vi "piezoDoubleWriteWriteFuncGen.vi"() -> (0 "success":bool)   [LabVIEW 2017]
doc: "Starts the piezo with a triangle or sine wave in continuous mode."
uses:
  <vilib>/DAQmx/write.llb/DAQmx Write (Analog 2D DBL NChan NSamp).vi
  globalDevices.vi
  globalUtilities.vi
  <vilib>/DAQmx/miscellaneous.llb/DAQmx Fill In Error Info.vi
panel:
  out "offset":dbl
  out "amplitude":dbl
  out "omega":dbl
  out "dt":dbl
  out "nT":i32
  out "Waveform Graph 4":dbl[](graph)
  out "Waveform Graph 3":dbl[](graph)
  out "used dt 2":dbl
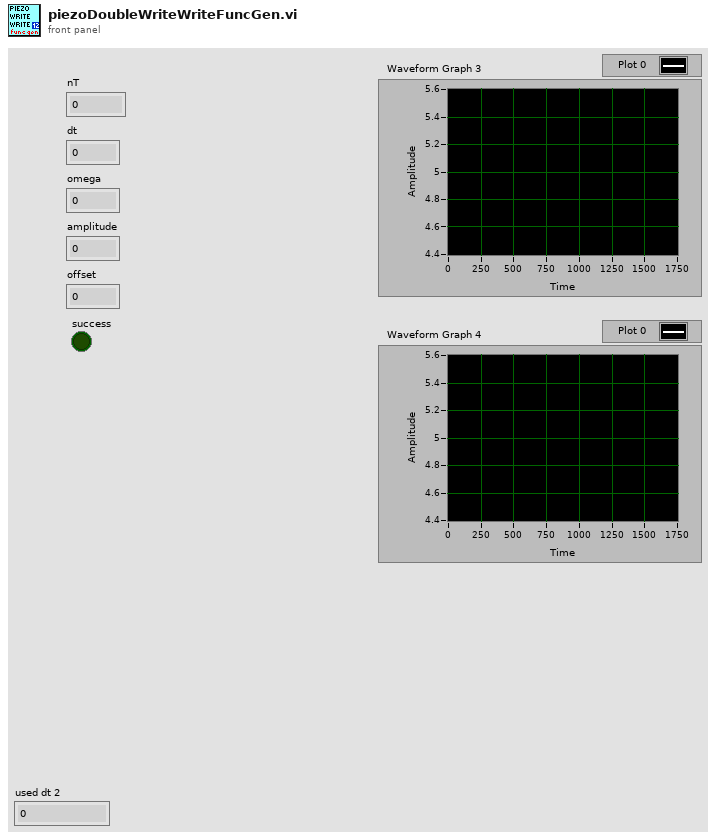
[diagram p1: front panel]
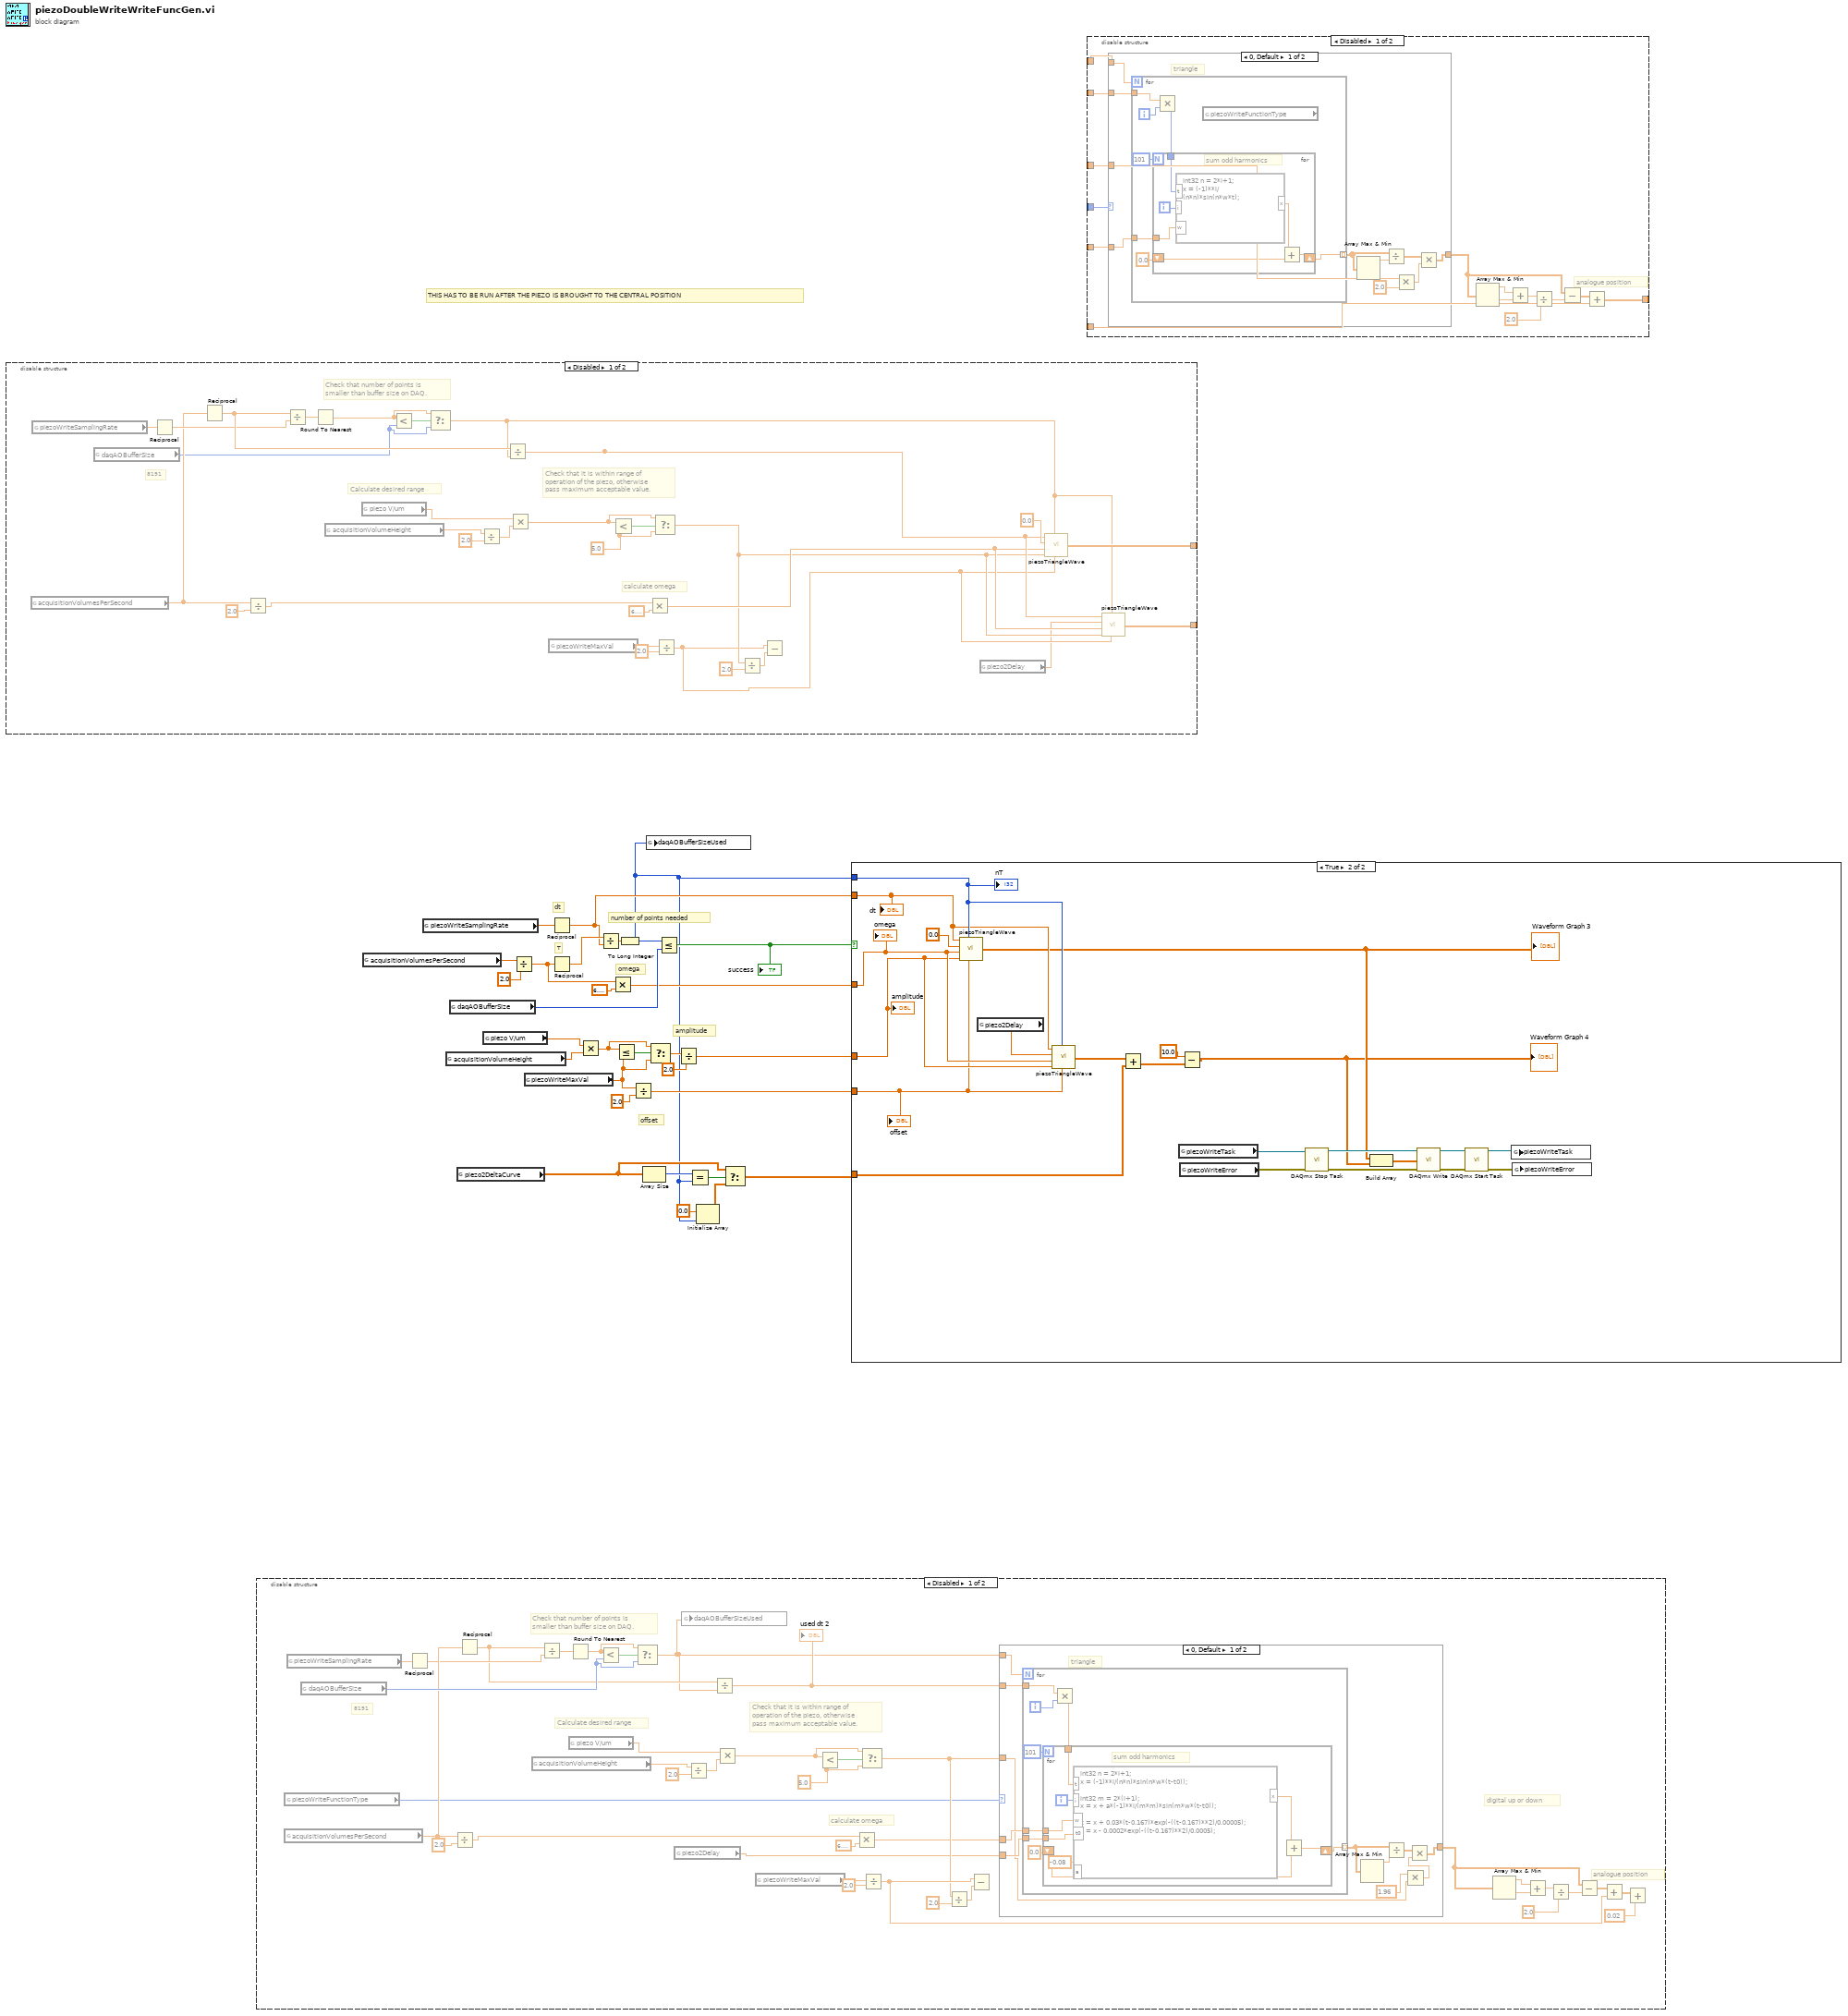
[diagram p0: block diagram]
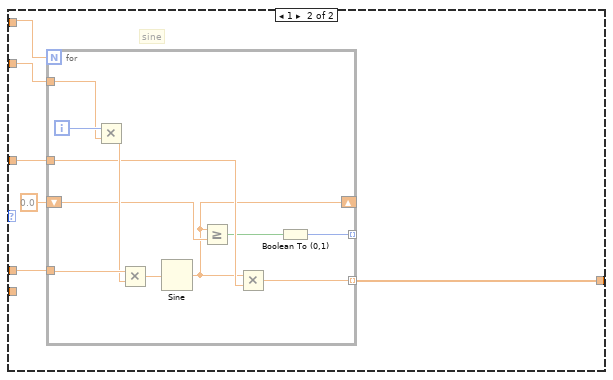
[diagram p4: hidden frame]
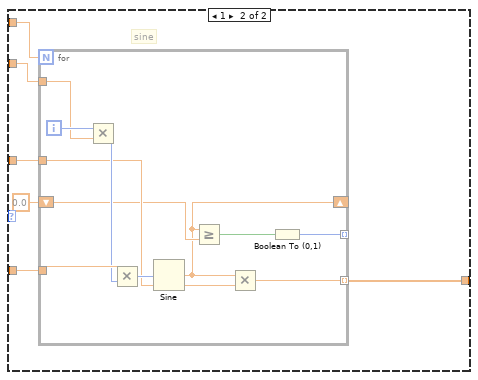
[diagram p6: hidden frame]
diagram:
  # "omega"
  # "amplitude"
  # "offset"
  # "number of points needed"
  # "T"
  # "dt"
  # "THIS HAS TO BE RUN AFTER THE PIEZO IS BROUGHT TO THE CENTRAL POSITION"
  n1 = disable-structure shown="Disabled" {
    disable-tunnel: [w38 _] -> _
    disable-tunnel: [w30 _] -> _
    frame Disabled {
      w53 = 5.0 ("y")
      # "8191"
      # "calculate omega"
      # "Check that number of points is\nsmaller than buffer size on DAQ."
      # "Check that it is within range of\noperation of the piezo, otherwise\npass maximum acceptable value."
      # "Calculate desired range"
      n2 = global read "globalUtilities.vi" "acquisitionVolumesPerSecond"() -> (w44:dbl)
      n3 = global read "globalDevices.vi" "piezoWriteSamplingRate"() -> (w48:dbl)
      n4 = global read "globalDevices.vi" "daqAOBufferSize"() -> (w41:i32)
      n5 = Reciprocal(x=w48) -> (1/x=w47:dbl)
      n6 = Reciprocal(x=w44) -> (1/x=w49:dbl)
      n7 = Divide(x=w44, y=2.0) -> (x/y=w42:dbl)
      n8 = Divide(x=w49, y=w47) -> (x/y=w51:dbl)
      n9 = Round To Nearest(number=w51) -> (nearest integer value=w29:dbl)
      n10 = global read "globalUtilities.vi" "acquisitionVolumeHeight"() -> (w58:dbl)
      n11 = global read "globalDevices.vi" "piezo V/um"() -> (w59:dbl)
      n12 = Less?(x=w29, y=w41) -> (x < y?=w50:bool)
      n13 = Select(t=w29, s=w50, f=w41) -> (s? t:f=w36:dbl)
      n14 = Divide(x=w58, y=2.0) -> (x/y=w56:dbl)
      n15 = Divide(x=w49, y=w36) -> (x/y=w35:dbl)
      n16 = Multiply(x=w59, y=w56) -> (x*y=w54:dbl)
      n17 = global read "globalDevices.vi" "piezoWriteMaxVal"() -> (w46:dbl)
      n18 = Less?(x=w54, y=w53) -> (x < y?=w55:bool)
      n19 = Multiply(x=w42, y=6.283185307179586) -> (x*y=w34:dbl)
      n20 = Select(t=w54, s=w55, f=w53) -> (s? t:f=w33:dbl)
      n21 = Divide(x=w46, y=2.0) -> (x/y=w32:dbl)
      n22 = Divide(x=w33, y=2.0) -> (x/y=w40:dbl)
      n23 = Subtract(x=w32, y=w40) -> ()  [unwired: 1 out]
      n24 = global read "globalDevices.vi" "piezo2Delay"() -> (w31:dbl)
      n25 = call "piezoTriangleWave.vi"("offset"=w32, "nT"=w36, "amplitude"=w33, "omega"=w34, "t0"=0.0, "dt"=w35) -> ("x+y"=w38:dbl[])
      n26 = call "piezoTriangleWave.vi"("offset"=w32, "nT"=w36, "amplitude"=w33, "omega"=w34, "t0"=w31, "dt"=w35) -> ("x+y"=w30:dbl[])
    }
    frame Enabled {
    }
  }
  n27 = disable-structure shown="Disabled" {
    frame Disabled {
      w70 = 5.0 ("y")
      # "8191"
      # "analogue position"
      # "digital up or down"
      # "calculate omega"
      # "Check that number of points is\nsmaller than buffer size on DAQ."
      # "Check that it is within range of\noperation of the piezo, otherwise\npass maximum acceptable value."
      # "Calculate desired range"
      n28 = global read "globalDevices.vi" "piezoWriteFunctionType"() -> (w82:u16)
      n29 = global read "globalUtilities.vi" "acquisitionVolumesPerSecond"() -> (w83:dbl)
      n30 = global read "globalDevices.vi" "piezoWriteSamplingRate"() -> (w78:dbl)
      n31 = global read "globalDevices.vi" "daqAOBufferSize"() -> (w86:i32)
      n32 = Reciprocal(x=w78) -> (1/x=w79:dbl)
      n33 = Divide(x=w83, y=2.0) -> (x/y=w85:dbl)
      n34 = Reciprocal(x=w83) -> (1/x=w76:dbl)
      n35 = global read "globalUtilities.vi" "acquisitionVolumeHeight"() -> (w65:dbl)
      n36 = Divide(x=w76, y=w79) -> (x/y=w73:dbl)
      n37 = Round To Nearest(number=w73) -> (nearest integer value=w75:dbl)
      n38 = global read "globalDevices.vi" "piezo V/um"() -> (w64:dbl)
      n39 = Less?(x=w75, y=w86) -> (x < y?=w74:bool)
      n40 = Select(t=w75, s=w74, f=w86) -> (s? t:f=w60:dbl)
      n41 = global read "globalDevices.vi" "piezo2Delay"() -> (w63:dbl)
      n42 = global write "globalDevices.vi" "daqAOBufferSizeUsed"(w60) -> ()
      n43 = Divide(x=w65, y=2.0) -> (x/y=w67:dbl)
      n44 = Divide(x=w76, y=w60) -> (x/y=w77:dbl)
      "used dt 2" <- w77
      n45 = Multiply(x=w64, y=w67) -> (x*y=w69:dbl)
      n46 = global read "globalDevices.vi" "piezoWriteMaxVal"() -> (w80:dbl)
      n47 = Less?(x=w69, y=w70) -> (x < y?=w68:bool)
      n48 = Multiply(x=w85, y=6.283185307179586) -> (x*y=w72:dbl)
      n49 = Select(t=w69, s=w68, f=w70) -> (s? t:f=w88:dbl)
      n50 = Divide(x=w80, y=2.0) -> (x/y=w97:dbl)
      n51 = Divide(x=w88, y=2.0) -> (x/y=w87:dbl)
      n52 = Subtract(x=w97, y=w87) -> ()  [unwired: 1 out]
      n53 = case shown="0, Default" w82 {
        tunnel: w72 -> [w106 w130]
        tunnel: w60 -> [w108 w129]
        tunnel: w77 -> [w107 w128]
        tunnel: w88 -> [w101 w127]
        tunnel: [w98 w125] -> w95
        tunnel: w63 -> [w105 _]
        frame 0, Default {
          # "triangle"
          n54 = for {
            N: w108 -> [_]
            tunnel: w107 -> [w116]
            tunnel: w106 -> [w113]
            tunnel: [w109] -> w102 mode=indexing
            tunnel: w105 -> [w110]
            i -> [w115]
            n55 = Multiply(x=w116, y=w115) -> (x*y=w112:dbl)
            n56 = for {
              N: 101 -> [_]
              tunnel: w113 -> [w122]
              tunnel: w112 -> [w124]
              shift-right: [w120] -> w109
              shift-left: 0.0 -> [w119]
              tunnel: w110 -> [w118]
              i -> [w123]
              # "sum odd harmonics"
              n57 = formula code="int32 n = 2*i+1;\nx = (-1)**i/(n*n)*sin(n*w*(t-t0));\n\nint32 m = 2*(i+1);\nx = x + a*(-1)**i/(m*m)*sin(m*w*(t-t0));\n\nx = x + 0.03*(t-0.167)*exp(-((t-0.167)**2)/0.00005);\nx = x - 0.0002*exp(-((t-0.167)**2)/0.0005);"("t"=w124, "i"=w123, "w"=w122, "t0"=w118, "a"=-0.08 ("input variable")) -> ("x"=w121:dbl)
              n58 = Add(x=w121, y=w119) -> (x+y=w120:dbl)
            }
          }
          n59 = Array Max & Min(array=w102) -> (max value=w104:dbl)  [unwired: 3 out]
          n60 = Divide(x=w102, y=w104) -> (x/y=w103:dbl[])
          n61 = Multiply(x=1.96, y=w101) -> (x*y=w99:dbl)
          n62 = Multiply(x=w103, y=w99) -> (x*y=w98:dbl[])
        }
        frame 1 {
          # "sine"
          n63 = for {
            N: w129 -> [_]
            tunnel: w130 -> [w141]
            tunnel: w128 -> [w139]
            tunnel: w127 -> [w136]
            tunnel: [w131] -> w125 mode=indexing
            shift-right: [w134] -> _
            shift-left: 0.0 -> [w135]
            tunnel: [w132] -> _ mode=indexing
            i -> [w140]
            n64 = Multiply(x=w140, y=w139) -> (x*y=w138:dbl)
            n65 = Multiply(x=w141, y=w138) -> (x*y=w137:dbl)
            n66 = Sine(x=w137) -> (sin(x)=w134:dbl)
            n67 = Greater Or Equal?(x=w134, y=w135) -> (x >= y?=w133:bool)
            n68 = Multiply(x=w134, y=w136) -> (x*y=w131:dbl)
            n69 = Boolean To (0,1)(Boolean=w133) -> (0, 1=w132:i16)
          }
        }
      }
      n70 = Array Max & Min(array=w95) -> (max value=w90:dbl, min value=w91:dbl)  [unwired: 2 out]
      n71 = Add(x=w90, y=w91) -> (x+y=w92:dbl)
      n72 = Divide(x=w92, y=2.0) -> (x/y=w94:dbl)
      n73 = Subtract(x=w95, y=w94) -> (x-y=w96:dbl[])
      n74 = Add(x=w96, y=w97) -> (x+y=w62:dbl[])
      n75 = Add(x=w62, y=0.02) -> ()  [unwired: 1 out]
    }
    frame Enabled {
    }
  }
  n76 = global read "globalUtilities.vi" "acquisitionVolumesPerSecond"() -> (w27:dbl)
  n77 = global read "globalDevices.vi" "piezoWriteSamplingRate"() -> (w28:dbl)
  n78 = global read "globalUtilities.vi" "acquisitionVolumeHeight"() -> (w21:dbl)
  n79 = global read "globalDevices.vi" "daqAOBufferSize"() -> (w24:i32)
  n80 = global read "globalDevices.vi" "piezo2DeltaCurve"() -> (w6:dbl[])
  n81 = global read "globalDevices.vi" "piezo V/um"() -> (w22:dbl)
  n82 = Divide(x=w27, y=2.0) -> (x/y=w11:dbl)
  n83 = global read "globalDevices.vi" "piezoWriteMaxVal"() -> (w18:dbl)
  n84 = Reciprocal(x=w28) -> (1/x=w9:dbl)
  n85 = Reciprocal(x=w11) -> (1/x=w25:dbl)
  n86 = Multiply(x=w22, y=w21) -> (x*y=w19:dbl)
  n87 = Divide(x=w25, y=w9) -> (x/y=w2:dbl)
  n88 = Multiply(x=w11, y=6.283185307179586) -> (x*y=w10:dbl)
  n89 = Less Or Equal?(x=w19, y=w18) -> (x <= y?=w20:bool)
  n90 = To Long Integer(number=w2) -> (32bit integer=w1:i32)
  n91 = Divide(x=w18, y=2.0) -> (x/y=w13:dbl)
  n92 = Array Size(array=w6) -> (size(s)=w8:i32)
  n93 = global write "globalDevices.vi" "daqAOBufferSizeUsed"(w1) -> ()
  n94 = Select(t=w19, s=w20, f=w18) -> (s? t:f=w16:dbl)
  n95 = Less Or Equal?(x=w1, y=w24) -> (x <= y?=w23:bool)
  "success" <- w23
  n96 = Divide(x=w16, y=2.0) -> (x/y=w14:dbl)
  n97 = Equal?(x=w8, y=w1) -> (x = y?=w7:bool)
  n98 = Initialize Array(0.0 ("element"), w1) -> (w4:dbl[])
  n99 = Select(t=w6, s=w7, f=w4) -> (s? t:f=w3:dbl[])
  n100 = case shown="True" w23 {
    tunnel: w14 -> [_ w158]
    tunnel: w13 -> [_ w157]
    tunnel: w10 -> [_ w159]
    tunnel: w1 -> [_ w162]
    tunnel: w9 -> [_ w161]
    tunnel: w3 -> [_ w145]
    frame False {
    }
    frame True {
      n101 = call "piezoTriangleWave.vi"("offset"=w157, "nT"=w162, "amplitude"=w158, "omega"=w159, "t0"=0.0, "dt"=w161) -> ("x+y"=w148:dbl[])
      "Waveform Graph 3" <- w148
      n102 = global read "globalDevices.vi" "piezo2Delay"() -> (w160:dbl)
      n103 = call "piezoTriangleWave.vi"("offset"=w157, "nT"=w162, "amplitude"=w158, "omega"=w159, "t0"=w160, "dt"=w161) -> ("x+y"=w149:dbl[])
      n104 = Add(x=w149, y=w145) -> (x+y=w144:dbl[])
      n105 = global read "globalDevices.vi" "piezoWriteTask"() -> (w147:refnum<k21>)
      n106 = global read "globalDevices.vi" "piezoWriteError"() -> (w146:errorcluster)
      n107 = Subtract(x=10.0, y=w144) -> (x-y=w143:dbl[])
      "Waveform Graph 4" <- w143
      n108 = call <vilib>:"DAQmx Stop Task.vi"("task/channels in"=w147, "error in"=w146) -> ("task out"=w150:refnum<k21>, "error out"=w151:errorcluster)  [unwired: 12 in]
      n109 = Build Array(w148, w143) -> (w156:dbl[][])
      n110 = call-poly <vilib>:"DAQmx Write.vi"("task/channels in"=w150, "data"=w156, "error in"=w151) -> ("task out"=w154:refnum<k21>, "error out"=w155:errorcluster)  [unwired: 10 in, 1 out]
      n111 = call <vilib>:"DAQmx Start Task.vi"("task/channels in"=w154, "error in"=w155) -> ("task out"=w152:refnum<k21>, "error out"=w153:errorcluster)  [unwired: 12 in]
      n112 = global write "globalDevices.vi" "piezoWriteTask"(w152) -> ()
      n113 = global write "globalDevices.vi" "piezoWriteError"(w153) -> ()
      "nT" <- w162
      "dt" <- w161
      "omega" <- w159
      "amplitude" <- w158
      "offset" <- w157
    }
  }
  n114 = disable-structure shown="Disabled" {
    disable-tunnel: _ -> [w177 _]
    disable-tunnel: [w169 _] -> _
    disable-tunnel: _ -> [w168 _]
    disable-tunnel: _ -> [w167 _]
    disable-tunnel: _ -> [w166 _]
    disable-tunnel: _ -> [w165 _]
    disable-tunnel: _ -> [w164 _]
    frame Disabled {
      # "analogue position"
      n115 = case shown="0, Default" w177 {
        tunnel: w166 -> [w185 w206]
        tunnel: w168 -> [w187 w205]
        tunnel: w167 -> [w186 w204]
        tunnel: w165 -> [w182 w203]
        tunnel: [w178 w202] -> w171
        frame 0, Default {
          # "triangle"
          n116 = for {
            N: w187 -> [_]
            tunnel: w186 -> [w194]
            tunnel: w185 -> [w191]
            tunnel: [w188] -> w183 mode=indexing
            i -> [w193]
            n117 = Multiply(x=w194, y=w193) -> (x*y=w190:i32)
            n118 = for {
              N: 101 -> [_]
              tunnel: w191 -> [w198]
              tunnel: w190 -> [w200]
              shift-right: [w196] -> w188
              shift-left: 0.0 -> [w195]
              i -> [w199]
              # "sum odd harmonics"
              n119 = formula code="int32 n = 2*i+1;\nx = (-1)**i/(n*n)*sin(n*w*t);"("t"=w200, "i"=w199, "w"=w198) -> ("x"=w197:dbl)
              n120 = Add(x=w197, y=w195) -> (x+y=w196:dbl)
            }
            n121 = global read "globalDevices.vi" "piezoWriteFunctionType"() -> ()  [unwired: 1 out]
          }
          n122 = Array Max & Min(array=w183) -> (max value=w184:dbl)  [unwired: 3 out]
          n123 = Divide(x=w183, y=w184) -> (x/y=w180:dbl[])
          n124 = Multiply(x=w182, y=2.0) -> (x*y=w179:dbl)
          n125 = Multiply(x=w180, y=w179) -> (x*y=w178:dbl[])
        }
        frame 1 {
          # "sine"
          n126 = for {
            N: w205 -> [_]
            tunnel: w206 -> [w217]
            tunnel: w204 -> [w215]
            tunnel: w203 -> [w212]
            tunnel: [w207] -> w202 mode=indexing
            shift-right: [w210] -> _
            shift-left: 0.0 -> [w211]
            tunnel: [w208] -> _ mode=indexing
            i -> [w216]
            n127 = Multiply(x=w216, y=w215) -> (x*y=w214:i32)
            n128 = Multiply(x=w217, y=w214) -> (x*y=w213:i32)
            n129 = Sine(x=w213) -> (sin(x)=w210:dbl)
            n130 = Greater Or Equal?(x=w210, y=w211) -> (x >= y?=w209:bool)
            n131 = Multiply(x=w210, y=w212) -> (x*y=w207:dbl)
            n132 = Boolean To (0,1)(Boolean=w209) -> (0, 1=w208:i16)
          }
        }
      }
      n133 = Array Max & Min(array=w171) -> (max value=w176:dbl, min value=w175:dbl)  [unwired: 2 out]
      n134 = Add(x=w176, y=w175) -> (x+y=w174:dbl)
      n135 = Divide(x=w174, y=2.0) -> (x/y=w172:dbl)
      n136 = Subtract(x=w171, y=w172) -> (x-y=w170:dbl[])
      n137 = Add(x=w170, y=w164) -> (x+y=w169:dbl[])
    }
    frame Enabled {
    }
  }
